vi "FPGA-Referense.vi"() -> ()   [LabVIEW 2019]
panel:
  in  "FPGA VI Reference":refnum<k20>
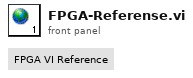
[diagram p1: front panel]
diagram:
